vi "Rotate Face 4.vi"(10 "Pretransform Rubix Array":T1[][](array[typedef]), 11 "Command":T2=-1 items=["Up"=-1, "Down"=1]) -> (1 "Axis":cluster{"X":sgl, "Y":sgl, "Z":sgl}={"X"=1.0, "Y"=0.0, "Z"=0.0}, 2 "Transform Rubix Array":T1[][](array[typedef]), 3 "Facets to move":T1[](array[typedef]))   [LabVIEW 2019]
uses:
  Rotate array command.ctl
  Rubix Array data type.ctl
  section movement.ctl
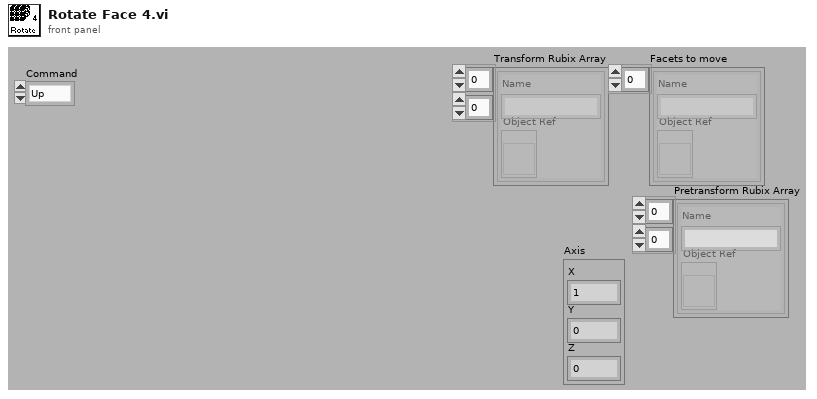
[diagram p1: front panel]
types:
  T1 = typedef "Rubix Array data type.ctl" = cluster{"Object Ref":refnum<vi>, "Name":string}
  T2 = typedef "Rotate array command.ctl" = i32
  T3 = typedef "section movement.ctl" = enum16{"Left", "Right"}
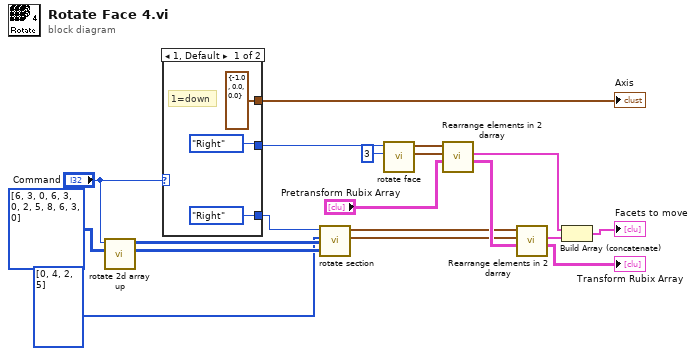
[diagram p0: block diagram]
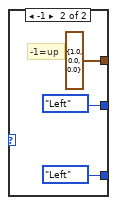
[diagram p2: hidden frame]
diagram:
  n1 = call "rotate 2d array up.vi"("From Facet"=i32[][] [[6, 3, 0], [6, 3, 0], [2, 5, 8], [6, 3, 0]], "Ring"="Command") -> ("Rotated"=w4:i32[][], "Dup Original"=w5:i32[][])  [unwired: 8 in]
  n2 = case shown="1, Default" "Command" {
    tunnel: [cluster{"X":sgl, "Y":sgl, "Z":sgl} {"X"=-1.0, "Y"=0.0, "Z"=0.0} ("Axis") cluster{"X":sgl, "Y":sgl, "Z":sgl} {"X"=1.0, "Y"=0.0, "Z"=0.0} ("Axis")] -> w12
    tunnel: [section_movement."Right" ("Direction") section_movement."Left" ("Direction")] -> w10
    tunnel: [section_movement."Right" ("Enum") section_movement."Left" ("Enum")] -> w8
    frame 1, Default {
      # "1=down"
    }
    frame -1 {
      # "-1=up"
    }
  }
  "Axis" <- w12
  n3 = call "rotate section.vi"("To Facet"=w4, "From Facet"=w5, "From"=i32[] [0, 4, 2, 5] ("From 2"), "Enum"=w8) -> ("To"=w6:cluster{"row":i32, "column":i32}[], "From"=w7:cluster{"row":i32, "column":i32}[])  [unwired: 6 in]
  n4 = call "rotate face.vi"("Face to act on"=3, "Direction"=w10) -> ("To"=w17:cluster{"row":i32, "column":i32}[], "From"=w18:cluster{"row":i32, "column":i32}[])  [unwired: 8 in]
  n5 = call "Rearrange elements in 2 darray.vi"("Pretransform Rubix Array"="Pretransform Rubix Array", "To"=w17, "From"=w18) -> ("Transform Rubix Array"=w13:T1[][], "Facets to move"=w19:T1[])  [unwired: 7 in]
  n6 = call "Rearrange elements in 2 darray.vi"("Pretransform Rubix Array"=w13, "To"=w6, "From"=w7) -> ("Transform Rubix Array"=→"Transform Rubix Array":T1[][], "Facets to move"=w15:T1[])  [unwired: 7 in]
  n7 = Build Array (concatenate)(w19, w15) -> (→"Facets to move":T1[])
